vi "benjamin_r - About.vi"   [LabVIEW 2017]
uses:
  vi.lib/addons/BenjaminR/shared/shared.lvlib
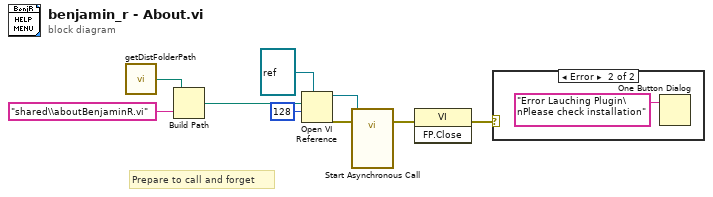
[diagram p0: block diagram]
diagram:
  # "Prepare to call and forget"
  n1 = call "getDistFolderPath.vi"() -> ("Dist Folder Path"=w1:path)
  n2 = Build Path(base path=w1, name or relative path="shared\\aboutBenjaminR.vi") -> (appended path=w4:path)
  n3 = Open VI Reference(type specifier VI Refnum (for type only)=refnum<vi> refnum ("VI Refnum"), vi path=w4, options=128) -> (vi reference=w8:refnum<vi>, error out=w6:errorcluster)  [unwired: 3 in]
  n4 = call-by-ref "Start Asynchronous Call"(reference=w8, error in=w6) -> (error out=w5:errorcluster)  [unwired: 1 in, 1 out]
  n5 = invoke class="VI" method="FP.Close"(error in=w5) -> (error out=w2:errorcluster)  [unwired: 2 in, 2 out]
  n6 = case shown="Error" w2 {
    frame No Error {
    }
    frame Error {
      n7 = One Button Dialog(message="Error Lauching Plugin\nPlease check installation") -> ()  [unwired: 1 in, 1 out]
    }
  }
